vi "ClassDataEditor.vi"(8 "error in (no error)":errorcluster, 10 "Experiment.lvclass":refnum<class "Experiment.lvclass">, 11 "Interface.lvclass":refnum<class "Interface.lvclass">) -> (0 "error out":errorcluster, 2 "Experiment.lvclass":refnum<class "Experiment.lvclass">, 3 "Interface.lvclass Out":refnum<class "Interface.lvclass">)   [LabVIEW 2019, in "Interface.lvclass"]
uses:
  Interface.lvclass
  Experiment Class/Experiment.lvclass
  Experiment Class/ClassCluster.ctl
  DevicesClass/BaseDevice/BaseDevice.lvclass
  DevicesClass/BaseDevice/BDClassCluster.ctl
  ItfDataCluster.ctl
  ScanParams.ctl
  CurveSetup.ctl
  2DGraphSetup.ctl
panel:
  in  "Interface Class":T1={"Experiment.lvclass"=refnum, "DataFileName"=path "", "HdrFileName"=path "", "DataFileRef"=refnum, "ScanParams"={"Entête"="", "Scan list"=[], "NbCourbe"=1, "IndCourbe"=0, "NomDon"=["RTêta;", "X&Y;"], "Session "=0, "Date"="", "Time"="", "VarParams"=[], "UserName"="", "ScanTableSize"=[], "VarPar list"=[], "DescKeyword"=""}, "DataQRefs"=[], "XYGraphCurves"=[], "AllCurves"=[], "CurvesParams"=[], "ScanGphInd"=[], "CurvesSetup"=[], "ScanDataQ"=[], "GraphRefArr"=[], "Graph_FA"=[], "FirstFreeFA"=0, "GraphConfig"=0, "PanRef"=refnum, "FAGraphNumArr"=[], "BaseDataPath"=path "", "ListBoxRef"=refnum, "VarParCount"=0, "GraphQRefArr"=[], "XScalesNames"=[], "YScalesNames"=[], "MainGraphQ"=refnum, "GraphEvent"=refnum, "2DGraphQRefArr"=[], "Scan2DGphInd"=[], "2DGraphRefArr"=[], "2DGphParams"=[], "GraphNumbers"=[], "LastGrphNum"=0, "AllDataQ"=[], "AllQRefs"=[], "VarParQRefs"=[], "DatQIndex"=[], "CalcQIndex"=[], "SubVarParQRefs"=[], "AllVarParQ"=[], "UseSubFolder"=FALSE}
  in  "BaseDev Data":T5={"Nom de ressource VISA"="", "DeviceCtrl"=[], "DataNames"=[], "ScanParamOut"=0.0, "HeaderString"="", "Functions"=[], "ScanFuncInd"=0, "Function"="", "StartStatPanel"=FALSE, "PanelVIRef"=refnum, "SubPanelRef"=refnum, "SubPanelCtrl"=[], "LoadedPanelIndex"=-1, "InstrumentName"="", "AvailFuncPan"=["ClassPanel"], "ScanTable"=[], "ScanPanelRef"=refnum, "ScanPanelPath"=path "", "Beforewait(ms)"=0, "Afterwait(ms)"=0, "SynchToClk(ms)"=-1, "FuncPanelIndex"=-1, "ClassQueue"=refnum, "ClassEvent"=refnum, "InstrParam"=[], "DatDisplayNm"=[], "ShowInstrNm"=[], "ShowParSuffix"=[], "ShowScanSuffix"=[], "ShowParValue"=[], "ParSuffix"=[], "ScanSuffix"=[], "Delta Time(ms)"=0, "BaseDataPath"=path "", "SubDatDisplayNm"=[], "SubScanTable(y)"=[], "SubVarParNm X"=[], "SubVarParNm Y"=[], "LastScanPos"=[]}
  in  "Experiment Data":T6
  in  "stop":bool
  in  "LoadedInst":i32
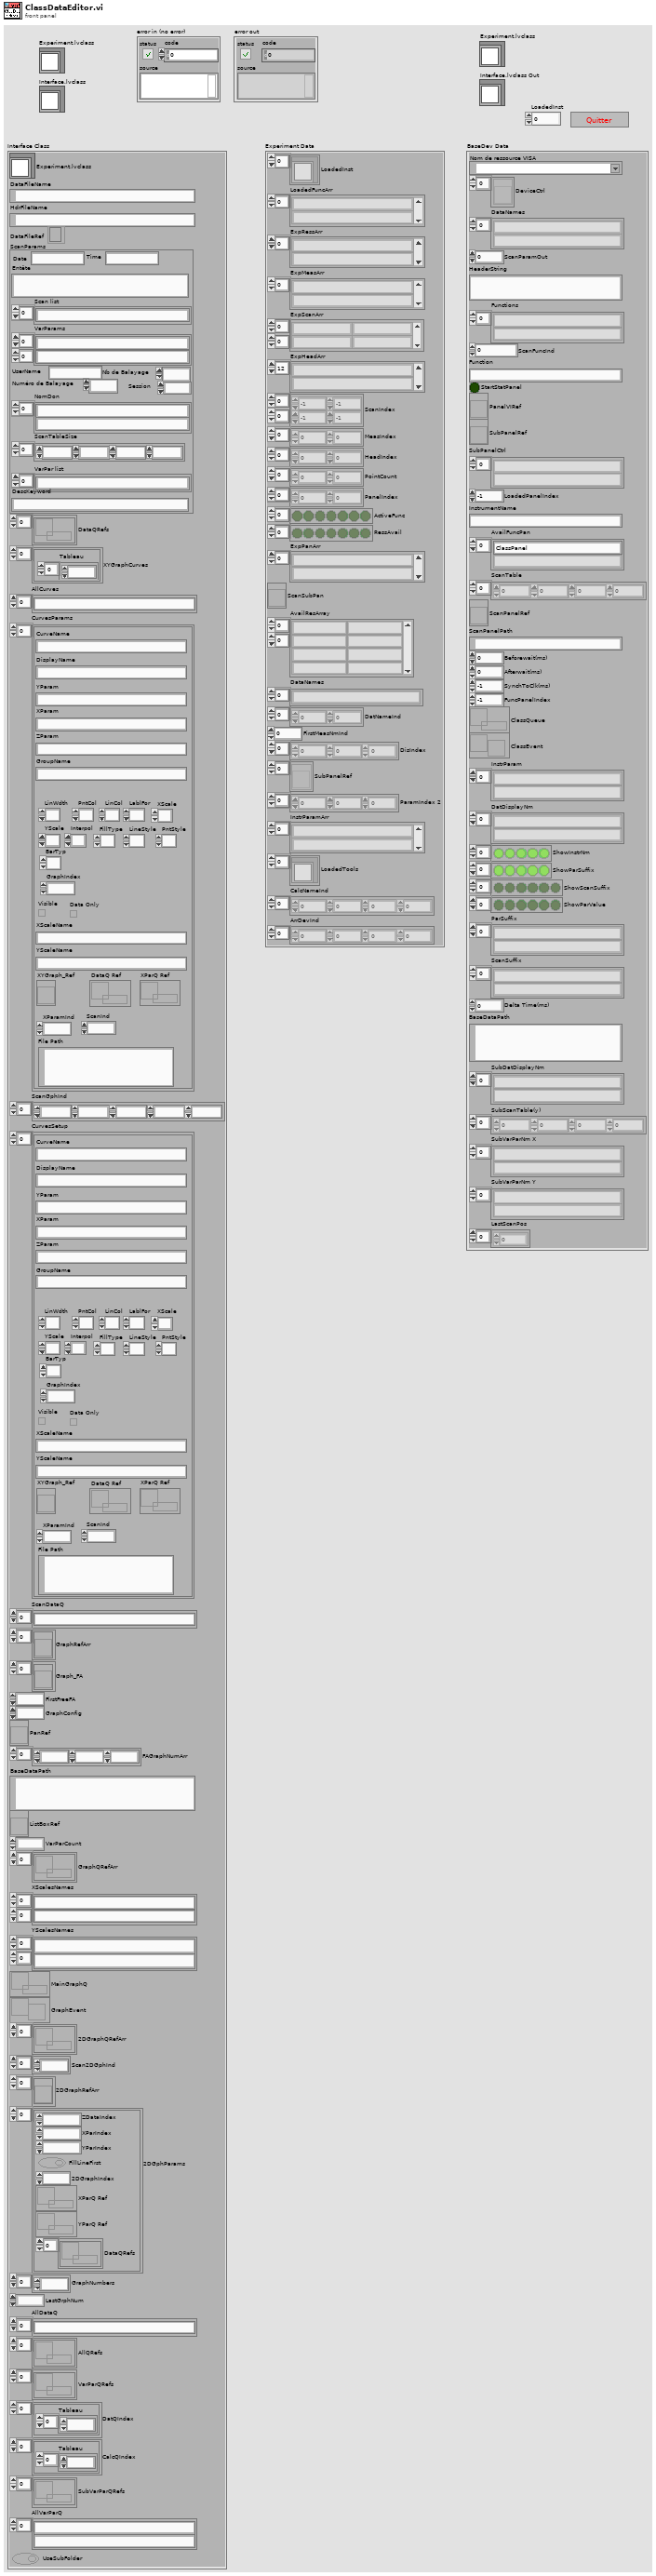
[diagram p1: front panel]
types:
  T1 = typedef "ItfDataCluster.ctl" = cluster{"Experiment.lvclass":refnum<class "Experiment.lvclass">, "DataFileName":path, "HdrFileName":path, "DataFileRef":refnum<file>, "ScanParams":T2, "DataQRefs":refnum<queue>[], "XYGraphCurves":cluster{"Tableau":i32[]}[], "AllCurves":string[], "CurvesParams":T3[], "ScanGphInd":i32[], "CurvesSetup":T3[], "ScanDataQ":string[], "GraphRefArr":refnum<vi>[], "Graph_FA":refnum<vi>[], "FirstFreeFA":u8, "GraphConfig":i32, "PanRef":refnum<vi>, "FAGraphNumArr":i32[], "BaseDataPath":path, "ListBoxRef":refnum<vi>, "VarParCount":i32, "GraphQRefArr":refnum<queue>[], "XScalesNames":string[][], "YScalesNames":string[][], "MainGraphQ":refnum<queue>, "GraphEvent":refnum<user-event>, "2DGraphQRefArr":refnum<queue>[], "Scan2DGphInd":i32[], "2DGraphRefArr":refnum<vi>[], "2DGphParams":T4[], "GraphNumbers":i32[], "LastGrphNum":i32, "AllDataQ":string[], "AllQRefs":refnum<queue>[], "VarParQRefs":refnum<queue>[], "DatQIndex":cluster{"Tableau":i32[]}[], "CalcQIndex":cluster{"Tableau":i32[]}[], "SubVarParQRefs":refnum<queue>[], "AllVarParQ":string[], "UseSubFolder":bool}
  T2 = typedef "Interface.lvclass/ScanParams.ctl" = cluster{"Entête":string, "Scan list":string[], "NbCourbe":i32, "IndCourbe":i64, "NomDon":string[], "Session ":i32, "Date":string, "Time":string, "VarParams":string[][], "UserName":string, "ScanTableSize":i32[], "VarPar list":string[], "DescKeyword":string}
  T3 = typedef "Interface.lvclass/CurveSetup.ctl" = cluster{"CurveName":string, "YParam":string, "XParam":string, "ZParam ":string, "GroupName":string, "LinWdth":u8, "PntCol":u32, "LinCol":u32, "LablFor":u8, "XScale":u32, "YScale":u32, "Interpol":u8, "DisplayName":string, "FillType":i16, "LineStyle":u8, "PntStyle":u8, "BarTyp":u8, "GraphIndex":i32, "Visible":bool, "XScaleName":string, "YScaleName":string, "XYGraph_Ref":refnum<vi>, "Data Only":bool, "DataQ Ref":refnum<queue>, "XParQ Ref":refnum<queue>, "XParamInd":i32, "ScanInd":i32, "File Path":path}
  T4 = typedef "2DGraphSetup.ctl" = cluster{"ZDataIndex":i32, "XParIndex":i32, "YParIndex":i32, "FillLineFirst":bool, "2DGraphIndex":i32, "XParQ Ref":refnum<queue>, "YParQ Ref":refnum<queue>, "DataQRefs":refnum<queue>[]}
  T5 = typedef "BDClassCluster.ctl" = cluster{"Nom de ressource VISA":refnum<visa-resource-name>, "DeviceCtrl":refnum<vi>[], "DataNames":string[], "ScanParamOut":dbl, "HeaderString":string, "Functions":string[], "ScanFuncInd":i32, "Function":string, "StartStatPanel":bool, "PanelVIRef":refnum<vi>, "SubPanelRef":refnum<vi>, "SubPanelCtrl":string[], "LoadedPanelIndex":i32, "InstrumentName":string, "AvailFuncPan":string[], "ScanTable":dbl[], "ScanPanelRef":refnum<vi>, "ScanPanelPath":path, "Beforewait(ms)":u32, "Afterwait(ms)":u32, "SynchToClk(ms)":i32, "FuncPanelIndex":i32, "ClassQueue":refnum<queue>, "ClassEvent":refnum<user-event>, "InstrParam":string[], "DatDisplayNm":string[], "ShowInstrNm":bool[], "ShowParSuffix":bool[], "ShowScanSuffix":bool[], "ShowParValue":bool[], "ParSuffix":string[], "ScanSuffix":string[], "Delta Time(ms)":u32, "BaseDataPath":path, "SubDatDisplayNm":string[], "SubScanTable(y)":dbl[], "SubVarParNm X":string[], "SubVarParNm Y":string[], "LastScanPos":dbl[]}
  T6 = typedef "ClassCluster.ctl" = cluster{"LoadedInst":refnum<class "BaseDevice.lvclass">[], "LoadedFuncArr":string[], "ExpRessArr":string[], "ExpMeasArr":string[], "ExpScanArr":string[][], "ExpHeadArr":string[], "ScanIndex":i32[][], "MeasIndex":i32[], "HeadIndex":i32[], "PointCount":i32[], "PanelIndex":i32[], "ActiveFunc":bool[], "RessAvail":bool[], "ExpPanArr":string[], "ScanSubPan":refnum<vi>, "AvailResArray":string[][], "DataNames":string[], "DatNameInd":i32[], "FirstMeasNmInd":i32, "DisIndex":i32[], "SubPanelRef":refnum<vi>[], "ParamIndex 2":i32[], "InstrParamArr":string[], "LoadedTools":refnum<class "BaseDevice.lvclass">[], "CalcNameInd":i32[], "ArrDevInd":i32[]}
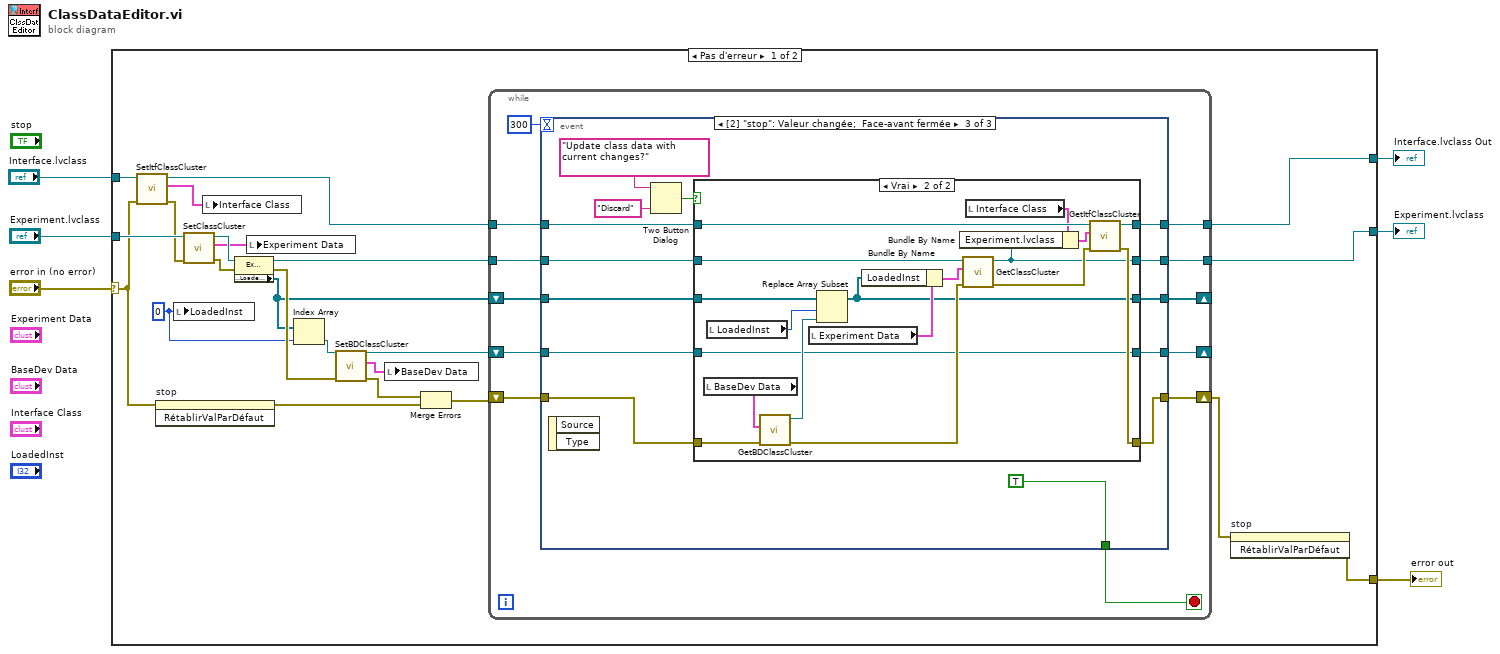
[diagram p0: block diagram]
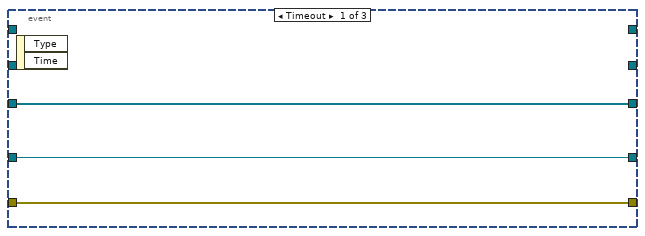
[diagram p2: hidden frame]
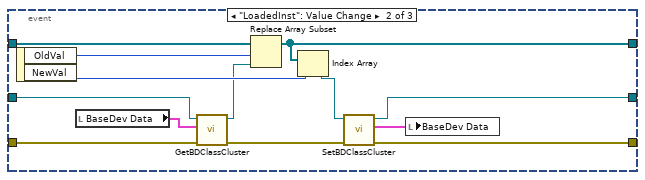
[diagram p3: hidden frame]
diagram:
  n1 = case shown="Pas d'erreur" "error in (no error)" {
    selector: "error in (no error)" -> [w8 w97]
    tunnel: "Experiment.lvclass" -> [w29 w96]
    tunnel: [w10 w97] -> w4
    tunnel: [w12 w96] -> w3
    tunnel: [w13 w95] -> w2
    tunnel: "Interface.lvclass" -> [w19 w95]
    frame No Error {
      w20 = 0 ("LoadedInst")
      n2 = call "SetItfClassCluster.vi"("error in (no error)"=w8, "Interface.lvclass"=w19) -> ("error out"=w15:errorcluster, "Interface Class"=w16:T1, "Interface.lvclass Out"=w17:refnum<class "Interface.lvclass">)  [unwired: 7 in]
      n3 = invoke on="stop" class="Bool" method="RétablirValParDéfaut"(error in=w8) -> (error out=w7:errorcluster)  [unwired: 2 in, 2 out]
      n4 = local write "LoadedInst"(w20) -> ()
      n5 = call "SetClassCluster.vi"("error in (no error)"=w15, "Experiment.lvclass"=w29) -> ("error out"=w27:errorcluster, "Experiment Data"=w23:T6, "Experiment.lvclass Out"=w26:refnum<class "Experiment.lvclass">)  [unwired: 7 in]
      n6 = local write "Interface Class"(w16) -> ()
      n7 = property class="Experiment.lvclass"(reference=w26, error in=w27) -> (reference out=w21:refnum<class "Experiment.lvclass">, error out=w22:errorcluster, "Accessor:LoadedInst"=w14:refnum<class "BaseDevice.lvclass">[])
      n8 = local write "Experiment Data"(w23) -> ()
      n9 = Index Array(array=w14, index=w20) -> (element=w25:refnum<class "BaseDevice.lvclass">)
      n10 = call "SetBDClassCluster.vi"("error in (no error)"=w22, "BaseDevice.lvclass"=w25) -> ("error out"=w28:errorcluster, "BaseDev Data"=w18:T5, "BaseDevice.lvclass Out"=w24:refnum<class "BaseDevice.lvclass">)  [unwired: 7 in]
      n11 = local write "BaseDev Data"(w18) -> ()
      n12 = Merge Errors(w28, w7) -> (w9:errorcluster)
      n13 = while {
        shift-right: [w37] -> w11
        shift-left: w9 -> [w39]
        tunnel: w21 -> [w33]
        tunnel: w17 -> [w32]
        shift-right: [w36] -> _
        shift-left: w14 -> [w40]
        shift-right: [w35] -> _
        shift-left: w24 -> [w38]
        tunnel: [w31] -> w13
        tunnel: [w30] -> w12
        stop <- w34 stop-if-true
        n14 = event shown="[2] \"stop\": Valeur changée;  Face-avant fermée" {
          selector: _ -> [_ _ _]
          dyn-events: _ -> [_ _ _]
          timeout: 300 -> [_ _ _]
          tunnel: w40 -> [w44 w57 w65]
          tunnel: w39 -> [w42 w53 w67]
          tunnel: w38 -> [w43 w52 w58]
          tunnel: [w42 w47 w66] -> w37
          tunnel: [w44 w46 w64] -> w36
          tunnel: [w43 w45 w59] -> w35
          tunnel: [_ _ TRUE] -> w34
          tunnel: w33 -> [_ _ w63]
          tunnel: w32 -> [_ _ w62]
          tunnel: [_ _ w61] -> w31
          tunnel: [_ _ w60] -> w30
          event Timeout {
            n15 = event-data() -> ()  [unwired: 1 in, 2 out]
          }
          event "LoadedInst": Value Change {
            n16 = event-data() -> ("OldVal"=w49:i32, "NewVal"=w56:i32)  [unwired: 1 in]
            n17 = local read "BaseDev Data"() -> (w51:T5)
            n18 = call "GetBDClassCluster.vi"("error in (no error)"=w53, "BaseDev Data"=w51, "BaseDevice.lvclass"=w52) -> ("error out"=w48:errorcluster, "BaseDevice.lvclass Out"=w50:refnum<class "BaseDevice.lvclass">)  [unwired: 7 in]
            n19 = Replace Array Subset(array=w57, new element=w50, index=w49) -> (w46:refnum<class "BaseDevice.lvclass">[])
            n20 = Index Array(array=w46, index=w56) -> (element=w55:refnum<class "BaseDevice.lvclass">)
            n21 = call "SetBDClassCluster.vi"("error in (no error)"=w48, "BaseDevice.lvclass"=w55) -> ("error out"=w47:errorcluster, "BaseDev Data"=w54:T5, "BaseDevice.lvclass Out"=w45:refnum<class "BaseDevice.lvclass">)  [unwired: 7 in]
            n22 = local write "BaseDev Data"(w54) -> ()
          }
          event "stop": Value Change; Panel Close {
            n23 = event-data() -> ()  [unwired: 1 in, 2 out]
            n24 = Two Button Dialog(message="Update class data with current changes?", 1:"Discard" ("F button name (\"Cancel\")")) -> (T button?=w69:bool)  [unwired: 1 in]
            n25 = case shown="Vrai" w69 {
              tunnel: w67 -> [w76 w92]
              tunnel: [w76 w84] -> w66
              tunnel: w65 -> [w73 w91]
              tunnel: [w73 w81] -> w64
              tunnel: w63 -> [w74 w89]
              tunnel: w62 -> [w75 w87]
              tunnel: [w75 w79] -> w61
              tunnel: [w74 w77] -> w60
              tunnel: [w72 w80] -> w59
              tunnel: w58 -> [w72 w80]
              frame False {
              }
              frame True {
                n26 = local read "BaseDev Data"() -> (w94:T5)
                n27 = local read "LoadedInst"() -> (w90:i32)
                n28 = call "GetBDClassCluster.vi"("error in (no error)"=w92, "BaseDev Data"=w94) -> ("error out"=w88:errorcluster, "BaseDevice.lvclass Out"=w93:refnum<class "BaseDevice.lvclass">)  [unwired: 8 in]
                n29 = local read "Experiment Data"() -> (w83:T6)
                n30 = Replace Array Subset(array=w91, new element=w93, index=w90) -> (w81:refnum<class "BaseDevice.lvclass">[])
                n31 = Bundle By Name(cluster=w83, "LoadedInst"=w81) -> (w82:T6)
                n32 = call "GetClassCluster.vi"("error in (no error)"=w88, "Experiment Data"=w82, "Experiment.lvclass"=w89) -> ("error out"=w85:errorcluster, "Experiment.lvclass Out"=w77:refnum<class "Experiment.lvclass">)  [unwired: 7 in]
                n33 = local read "Interface Class"() -> (w86:T1)
                n34 = Bundle By Name(cluster=w86, "Experiment.lvclass"=w77) -> (w78:T1)
                n35 = call "GetItfClassCluster.vi"("error in (no error)"=w85, "Interface Class"=w78, "Interface.lvclass"=w87) -> ("error out"=w84:errorcluster, "Interface.lvclass Out"=w79:refnum<class "Interface.lvclass">)  [unwired: 7 in]
              }
            }
          }
        }
      }
      n36 = invoke on="stop" class="Bool" method="RétablirValParDéfaut"(error in=w11) -> (error out=w10:errorcluster)  [unwired: 2 in, 2 out]
    }
    frame Error {
    }
  }
  "Interface.lvclass Out" <- w2
  "Experiment.lvclass" <- w3
  "error out" <- w4
